vi "Begin.vi"(8 "error in (no error)":errorcluster, 11 "Joysticks in":refnum<class "Joysticks.lvclass">) -> (0 "error out":errorcluster, 3 "Joysticks out":refnum<class "Joysticks.lvclass">)   [LabVIEW 2018, in "Joysticks.lvlib" / "Joysticks.lvclass"]
doc: "This VI is used to open the joystick control references."
uses:
  Joysticks.lvclass
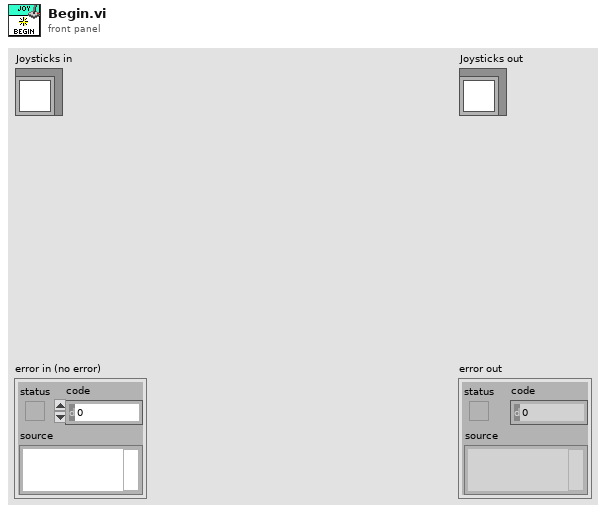
[diagram p1: front panel]
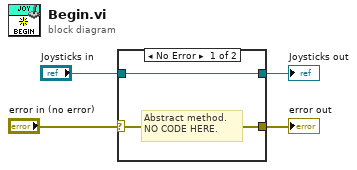
[diagram p0: block diagram]
diagram:
  n1 = case shown="No Error" "error in (no error)" {
    selector: "error in (no error)" -> [w5 w8]
    tunnel: [w5 w8] -> w3
    tunnel: [w6 w7] -> w1
    tunnel: "Joysticks in" -> [w6 w7]
    frame No Error {
      # "Abstract method.\nNO CODE HERE."
    }
    frame Error {
    }
  }
  "error out" <- w3
  "Joysticks out" <- w1
